vi "DriveBegin.vi"(8 "error in (no error)":errorcluster) -> (0 "error out":errorcluster)   [LabVIEW 2023]
doc: "Begin for Drive\n\nInputs:\n -- Error in -- Error cluster -- propagated error input\n\nOutputs:\n -- Error out -- Error cluster -- progated error output"
uses:
  <vilib>/Rock Robotics/WPI/ThirdParty/JAS_Junk/TrajLib/TypeDef/SWERVE_DRIVE_MODULE_POSITION.ctl
  <vilib>/Rock Robotics/WPI/ThirdParty/JAS_Junk/TrajLib/TypeDef/ROTATION2D.ctl
  DriveGlobal.vi
  <vilib>/Rock Robotics/WPI/ThirdParty/JAS_Junk/TrajLib/Trajectory_Library.lvlib
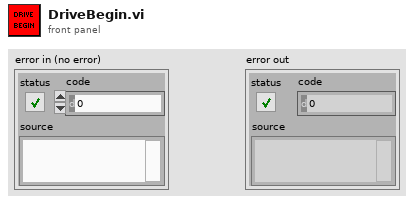
[diagram p1: front panel]
types:
  T1 = typedef "Trajectory_Library.lvlib/SWERVE_DRIVE_MODULE_POSITION.ctl" = cluster{"Distance":dbl, "Angle":T2, "P":bool}
  T2 = typedef "Trajectory_Library.lvlib/ROTATION2D.ctl" = cluster{"VALUE":dbl, "COS":dbl, "SIN":dbl}
  T3 = typedef "Trajectory_Library.lvlib/TRANSLATION2D.ctl" = cluster{"X":dbl, "Y":dbl}
  T4 = typedef "Trajectory_Library.lvlib/SWERVE_DRIVE_KINEMATICS.ctl" = cluster{"NumModules":i32, "InverseKinematics":T5, "ForwardKinematics":T5, "Modules":T3[], "PrevCoR":T3, "SavedModuleStates":T6[]}
  T5 = typedef "NI_Matrix.lvlib/RealMatrix.ctl" = dbl[][]
  T6 = typedef "Trajectory_Library.lvlib/SWERVE_DRIVE_MODULE_STATE.ctl" = cluster{"Speed":dbl, "Angle":T2}
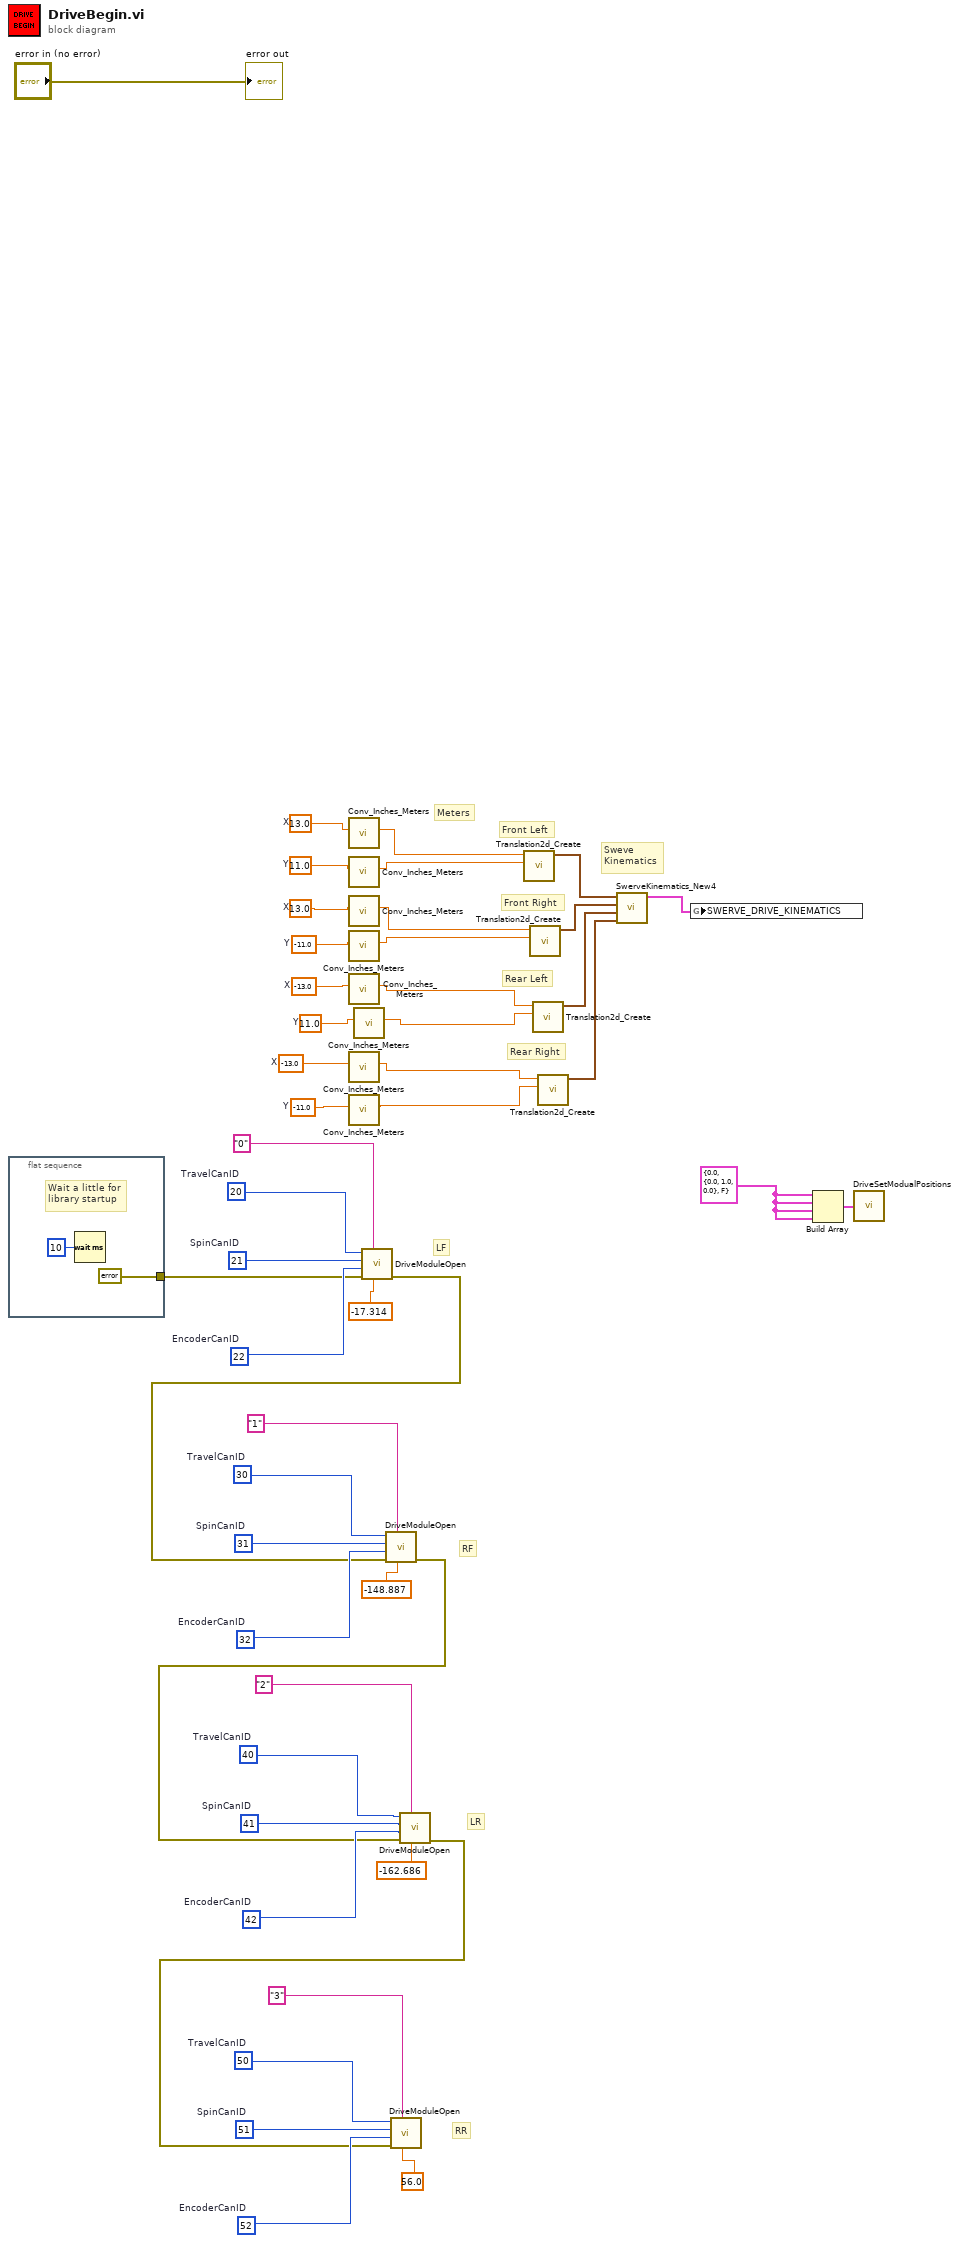
[diagram p0: block diagram]
diagram:
  w1 = T1 {"Distance"=0.0, "Angle"={"VALUE"=0.0, "COS"=1.0, "SIN"=0.0}, "P"=FALSE} ("SWERVE_DRIVE_MODULE_POSITION")
  w13 = u8 50  # TravelCanID
  w12 = u8 51  # SpinCanID
  w11 = u8 52  # EncoderCanID
  w16 = u8 40  # TravelCanID
  w15 = u8 41  # SpinCanID
  w14 = u8 42  # EncoderCanID
  w19 = u8 30  # TravelCanID
  w18 = u8 31  # SpinCanID
  w17 = u8 32  # EncoderCanID
  w20 = u8 20  # TravelCanID
  w21 = u8 21  # SpinCanID
  w22 = u8 22  # EncoderCanID
  w29 = -13.0  # X
  w28 = -11.0  # Y
  w31 = -13.0  # X
  w30 = 11.0  # Y
  w33 = 13.0  # X
  w32 = -11.0  # Y
  w35 = 13.0  # X
  w34 = 11.0  # Y
  # "RR"
  # "LR"
  # "RF"
  # "LF"
  # "Meters"
  # "Sweve\nKinematics"
  # "Rear Right"
  # "Rear Left"
  # "Front Right"
  # "Front Left"
  n1 = flat-sequence {
    tunnel: [errorcluster {"status"=FALSE, "code"=0, "source"=""} ("error in")] -> w3
    frame #0 {
      # "Wait a little for\nlibrary startup"
      n2 = Wait (ms)(milliseconds to wait=u32 10) -> ()  [unwired: 1 out]
    }
  }
  n3 = call <vilib>:"Conv_Inches_Meters.vi"("INCH"=w35) -> ("Meters"=w36:dbl)  [unwired: 10 in]
  n4 = call <vilib>:"Conv_Inches_Meters.vi"("INCH"=w34) -> ("Meters"=w37:dbl)  [unwired: 10 in]
  n5 = call <vilib>:"Conv_Inches_Meters.vi"("INCH"=w33) -> ("Meters"=w38:dbl)  [unwired: 10 in]
  n6 = call <vilib>:"Conv_Inches_Meters.vi"("INCH"=w32) -> ("Meters"=w39:dbl)  [unwired: 10 in]
  n7 = call <vilib>:"Conv_Inches_Meters.vi"("INCH"=w31) -> ("Meters"=w40:dbl)  [unwired: 10 in]
  n8 = call <vilib>:"Conv_Inches_Meters.vi"("INCH"=w29) -> ("Meters"=w43:dbl)  [unwired: 10 in]
  n9 = call <vilib>:"Conv_Inches_Meters.vi"("INCH"=w28) -> ("Meters"=w42:dbl)  [unwired: 10 in]
  n10 = call <vilib>:"Conv_Inches_Meters.vi"("INCH"=w30) -> ("Meters"=w41:dbl)  [unwired: 10 in]
  n11 = call "DriveModuleOpen.vi"("Magnet Offset (Degrees)"=-17.314, "ModualNamePrefix"="0", "error in"=w3, "EncoderCanID"=w22, "SpinCanID"=w21, "TravelCanID"=w20) -> ("error out"=w6:errorcluster)  [unwired: 5 in]
  n12 = call "DriveModuleOpen.vi"("Magnet Offset (Degrees)"=-148.887, "ModualNamePrefix"="1", "error in"=w6, "EncoderCanID"=w17, "SpinCanID"=w18, "TravelCanID"=w19) -> ("error out"=w5:errorcluster)  [unwired: 5 in]
  n13 = call "DriveModuleOpen.vi"("Magnet Offset (Degrees)"=-162.686, "ModualNamePrefix"="2", "error in"=w5, "EncoderCanID"=w14, "SpinCanID"=w15, "TravelCanID"=w16) -> ("error out"=w4:errorcluster)  [unwired: 5 in]
  n14 = call "DriveModuleOpen.vi"("Magnet Offset (Degrees)"=56.0, "ModualNamePrefix"="3", "error in"=w4, "EncoderCanID"=w11, "SpinCanID"=w12, "TravelCanID"=w13) -> ()  [unwired: 5 in, 1 out]
  n15 = call <vilib>:"Translation2d_Create.vi"("Y"=w37, "X"=w36) -> ("TRANSLATION"=w44:T3)  [unwired: 9 in]
  n16 = call <vilib>:"Translation2d_Create.vi"("Y"=w39, "X"=w38) -> ("TRANSLATION"=w45:T3)  [unwired: 9 in]
  n17 = call <vilib>:"Translation2d_Create.vi"("Y"=w41, "X"=w40) -> ("TRANSLATION"=w46:T3)  [unwired: 9 in]
  n18 = call <vilib>:"Translation2d_Create.vi"("Y"=w42, "X"=w43) -> ("TRANSLATION"=w47:T3)  [unwired: 9 in]
  n19 = call <vilib>:"SwerveKinematics_New4.vi"("wheel 3"=w47, "wheel 2"=w46, "wheel 1"=w45, "wheel 0"=w44) -> ("SWERVE_DRIVE_KINEMATICS"=w27:T4)  [unwired: 7 in]
  n20 = global write "DriveGlobal.vi" "SWERVE_DRIVE_KINEMATICS"(w27) -> ()
  n21 = Build Array(w1, w1, w1, w1) -> (w2:T1[])
  n22 = call "DriveSetModualPositions.vi"("Swerve_Drive_Modual_Position"=w2) -> ()  [unwired: 11 in]
  "error out" <- "error in (no error)"
